vi "FullAlign.vi"(0 "Joystick 0":dbl, 5 "Joystick 1":dbl, 7 "Distance":dbl, 9 "Angle":dbl, 11 "Button":bool=TRUE) -> (4 "Right Motor":dbl, 6 "Left Motor":dbl, 12 "Greater":bool, 13 "In Range?":bool, 14 "Less than":bool)   [LabVIEW 2016]
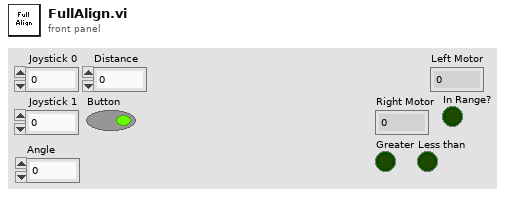
[diagram p1: front panel]
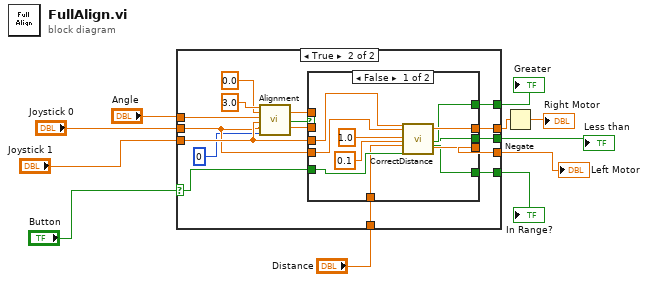
[diagram p0: block diagram]
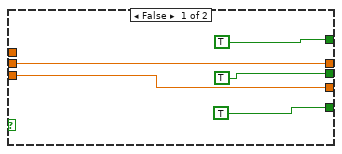
[diagram p2: hidden frame]
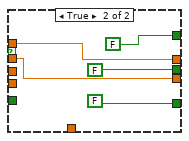
[diagram p3: hidden frame]
diagram:
  n1 = case shown="True" "Button" {
    selector: "Button" -> [_ w22]
    tunnel: "Joystick 1" -> [w15 w27]
    tunnel: "Joystick 0" -> [w16 w26]
    tunnel: [w15 w32] -> w1
    tunnel: [w16 w31] -> w3
    tunnel: "Angle" -> [_ w29]
    tunnel: [TRUE w21] -> w7
    tunnel: [TRUE w20] -> w6
    tunnel: [TRUE w19] -> w8
    tunnel: "Distance" -> [_ w18]
    frame False {
    }
    frame True {
      n2 = call "Alignment.vi"("Range"=3.0, "Target"=0.0, "Gyroscope Angle"=w29, "RightMotorSpeed"=w27, "LeftMotorSpeed"=w26, "POV"=0) -> ("Right Motor"=w25:dbl, "LeftAndRight?"=w23:bool, "Left Motor"=w24:dbl)  [unwired: 11 in]
      n3 = case shown="False" w23 {
        tunnel: w27 -> [w39 _]
        tunnel: w26 -> [w40 _]
        tunnel: [w38 w47] -> w32
        tunnel: [w37 w48] -> w31
        tunnel: w22 -> [w41 _]
        tunnel: w25 -> [_ w48]
        tunnel: w24 -> [_ w47]
        tunnel: [w36 FALSE] -> w21
        tunnel: [w35 FALSE] -> w20
        tunnel: [w34 FALSE] -> w19
        tunnel: w18 -> [w33 _]
        frame False {
          n4 = call "CorrectDistance.vi"("JoyStick 1"=w39, "JoyStick 2"=w40, "CenterPoint"=1.0, "Range"=0.1, "Distance"=w33, "Button"=w41) -> ("Right Motor"=w37:dbl, "Left Motor"=w38:dbl, "Less than"=w35:bool, "Greater"=w36:bool, "In Range?"=w34:bool)  [unwired: 16 in, 1 out]
        }
        frame True {
        }
      }
    }
  }
  "Left Motor" <- w1
  "In Range?" <- w8
  "Greater" <- w7
  "Less than" <- w6
  n5 = Negate(x=w3) -> (-x=→"Right Motor":dbl)
